vi "V3Test1.vi"   [LabVIEW 2019]
uses:
  Downloads/V3PKLIBTest/WSCbot_V3_Toolkit.lvlibp
types:
  T1 = cluster{"proportional gain (Kc)":dbl, "integral time (Ti, min)":dbl, "derivative time (Td, min)":dbl}
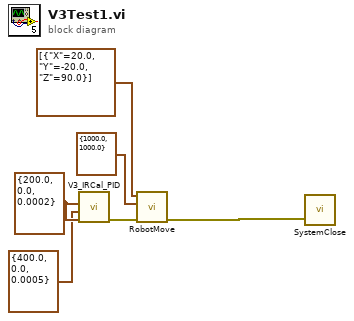
[diagram p0: block diagram]
diagram:
  w2 = T1 {"proportional gain (Kc)"=200.0, "integral time (Ti, min)"=0.0, "derivative time (Td, min)"=0.0002} ("PID gains")
  n1 = call "V3_IRCal_PID.vi"("PID gains 3"=w2, "PID gains 2"=T1 {"proportional gain (Kc)"=400.0, "integral time (Ti, min)"=0.0, "derivative time (Td, min)"=0.0005}, "PID gains"=w2) -> ("error out"=w5:errorcluster)  [unwired: 8 in]
  n2 = call "RobotMove.vi"("error in (no error)"=w5, "Speed/ACC"=cluster{dbl, dbl} {1000.0, 1000.0}, "XYZ"=cluster{"X":dbl, "Y":dbl, "Z":dbl}[] [{"X"=20.0, "Y"=-20.0, "Z"=90.0}]) -> ("error out"=w4:errorcluster)  [unwired: 8 in]
  n3 = call "SystemClose.vi"("error in"=w4) -> ()  [unwired: 2 in, 1 out]
